vi "Do.vi"(8 "error in":errorcluster, 10 "Actor in":refnum<class "Actor.lvclass">, 11 "Reply Msg DS in":refnum<class "Reply Msg DataSocket Connections Managed.lvclass">) -> (0 "error out":errorcluster, 2 "Actor out":refnum<class "Actor.lvclass">)   [LabVIEW 2023, in "Reply Msg DataSocket Connections Managed.lvclass"]
uses:
  Reply Msg DataSocket Connections Managed.lvclass
  Reply Msg DataSocket Connections Managed.lvclass/Reply Msg DataSocket Connections Managed.ctl
  <vilib>/ActorFramework/Actor/Actor.lvclass
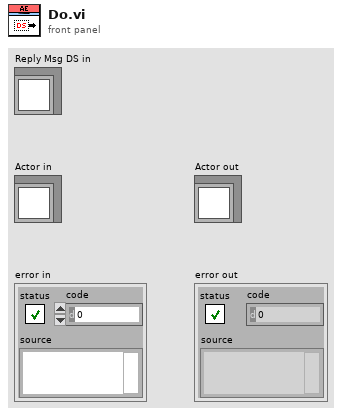
[diagram p1: front panel]
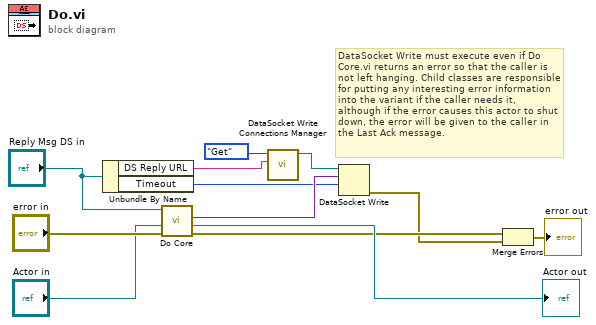
[diagram p0: block diagram]
diagram:
  # "DataSocket Write must execute even if Do Core.vi returns an error so that the caller is not left hanging. Child classes are responsible for putting any interesting error information into the variant if the caller needs it, although if the error causes this actor to shut down, the error will be given to the caller in the Last Ack message."
  n1 = Unbundle By Name("Reply Msg DS in") -> ("DS Reply URL"=w1:string, "Timeout"=w4:i32)
  n2 = call-dynamic "Do Core.vi"("error in"="error in", "Actor in"="Actor in", "Reply Msg DS in"="Reply Msg DS in") -> ("error out"=w8:errorcluster, "Actor out"=→"Actor out":refnum<class "Actor.lvclass">, "Reply"=w5:variant)  [unwired: 6 in]
  n3 = call "DataSocket Write Connections Manager.vi"("URL"=w1, "Action"=enum16{"Get", "Close", "Close All"}."Get") -> ("connection id"=w3:refnum<k13>)  [unwired: 9 in]
  n4 = DataSocket Write(9:w4, 10:w5, 11:w3) -> (0:w6:errorcluster)  [unwired: 1 in, 2 out]
  n5 = Merge Errors(w8, w6) -> (→"error out":errorcluster)
